vi "SQLite Query - Add New Columns.vi"(8 "error in (no error)":errorcluster, 9 "LV Data Types":T1[](array[typedef]) format="%.0x", 10 "Headers":string[](array[string]), 11 "TableLogger_SQLite_Actor in":refnum<class "TableLogger_SQLite_Actor.lvclass">) -> (0 "error out":errorcluster, 3 "TableLogger_SQLite_Actor out":refnum<class "TableLogger_SQLite_Actor.lvclass">)   [LabVIEW 2014, in "TableLogger_SQLite_Actor.lvlib" / "TableLogger_SQLite_Actor.lvclass"]
uses:
  TableLogger_SQLite_Actor.lvclass
  <userlib>/_OpenG.lib/lvdata/lvdata.llb/Type Descriptor Enumeration__ogtk.ctl
  TableLogger_SQLite_Actor.lvclass/TableLogger_SQLite_Actor.ctl
  <vilib>/drjdpowell/SQLite Library/SQL Connection/Execute SQL.vi
  <userlib>/_OpenG.lib/array/array.llb/Remove Duplicates from 1D Array (String)__ogtk.vi
  <vilib>/drjdpowell/SQLite Library/SQL Connection/Execute SQL (No results).vi
  <vilib>/drjdpowell/SQLite Library/SQLite.lvlib
  <vilib>/drjdpowell/SQLite Library/SQL Connection/Connection.lvclass
panel:
  # "Connector Pane"
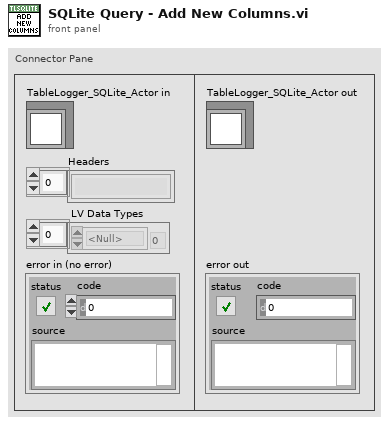
[diagram p1: front panel]
types:
  T1 = typedef "Type Descriptor Enumeration__ogtk.ctl" = enum8{"<Null>", "I8", "I16", "I32", "I64", "U8", "U16", "U32", "U64", "SGL", "DBL", "EXT", "CSG", "CDB", "CXT", "0x0F", "0x10", "0x11", "0x12", "0x13", "0x14", "Enum U8", "Enum U16", "Enum U32", "Enum U64", "SGL PQ", "DBL PQ", "EXT PQ", "CSG PQ", "CDB PQ", "CXT PQ", "0x1F", "0x20", "Boolean", "0x22", "0x23", "0x24", "0x25", "0x26", "0x27", "0x28", "0x29", "0x2A", "0x2B", "0x2C", "0x2D", "0x2E", "0x2F", "String", "0x31", "Path", "Pict", "0x34", "0x35", "0x36", "DAQ", "0x38", "0x39", "0x3A", "0x3B", "0x3C", "0x3D", "0x3E", "0x3F", "Array", "0x41", "0x42", "0x43", "0x44", "0x45", "0x46", "0x47", "0x48", "0x49", "0x4A", "0x4B", "0x4C", "0x4D", "0x4E", "0x4F", "Cluster", "0x51", "0x52", "Variant", "Waveform", "0x55", "0x56", "0x57", "0x58", "0x59", "0x5A", "0x5B", "0x5C", "0x5D", "0x5E", "0x5F", "0x60", "0x61", "0x62", "0x63", "0x64", "0x65", "0x66", "0x67", "0x68", "0x69", "0x6A", "0x6B", "0x6C", "0x6D", "0x6E", "0x6F", "Refnum"}
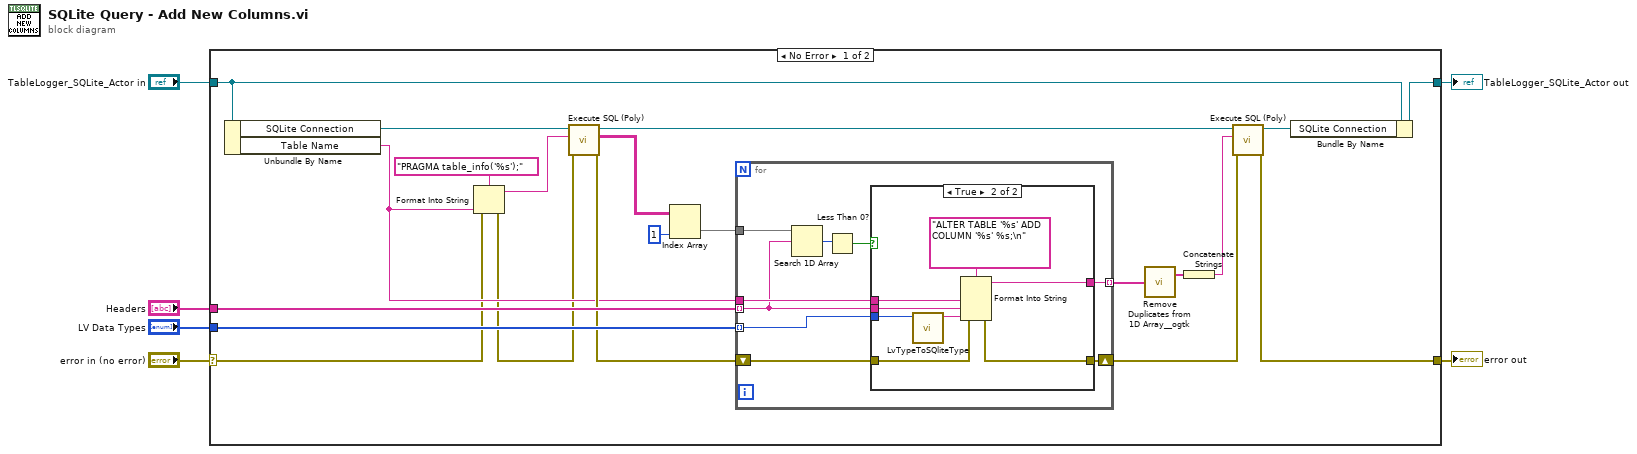
[diagram p0: block diagram]
diagram:
  n1 = case shown="No Error" "error in (no error)" {
    selector: "error in (no error)" -> [w9 w46]
    tunnel: [w26 w47] -> w5
    tunnel: "Headers" -> [w23 _]
    tunnel: "LV Data Types" -> [w21 _]
    tunnel: [w12 w46] -> w4
    tunnel: "TableLogger_SQLite_Actor in" -> [w11 w47]
    frame No Error {
      n2 = Unbundle By Name(w11) -> ("SQLite Connection"=w18:refnum<class "Connection.lvclass">, "Table Name"=w10:string)
      n3 = Format Into String(format string="PRAGMA table_info('%s');" ("SQL"), error in=w9, w10) -> (resulting string=w14:string, error out=w8:errorcluster)  [unwired: 1 in]
      n4 = call-poly <vilib>:"Execute SQL (Poly).vi"("error in (no error)"=w8, "SQL"=w14, "SQLite Connection in"=w18) -> ("error out"=w19:errorcluster, "Result Set"=w15:string[][], "SQLite Connection"=w7:refnum<class "Connection.lvclass">)  [unwired: 5 in, 1 out]
      n5 = Index Array(array=w15, index (col)=1 ("disabled index (col)")) -> (element=w17:string[])  [unwired: 1 in]
      n6 = for {
        tunnel: w17 -> [w36]
        tunnel: w10 -> [w32]
        tunnel: w23 -> [w31] mode=indexing
        shift-right: [w34] -> w20
        shift-left: w19 -> [w35]
        tunnel: w21 -> [w29] mode=indexing
        tunnel: [w28] -> w24 mode=indexing
        n7 = Search 1D Array(1D array=w36, element=w31) -> (index of element=w33:i32)  [unwired: 1 in]
        n8 = Less Than 0?(x=w33) -> (x < 0?=w30:bool)
        n9 = case shown="True" w30 {
          tunnel: w35 -> [w37 w40]
          tunnel: [w37 w39] -> w34
          tunnel: w32 -> [_ w44]
          tunnel: w31 -> [_ w43]
          tunnel: w29 -> [_ w42]
          tunnel: [_ w41] -> w28
          frame False {
          }
          frame True {
            n10 = call "LvTypeToSQliteType.vi"("Type Descriptor Enumeration"=w42) -> ("String"=w38:string)  [unwired: 10 in]
            n11 = Format Into String(format string="ALTER TABLE '%s' ADD COLUMN '%s' %s;\n" ("SQL"), error in=w40, w44, w43, w38) -> (resulting string=w41:string, error out=w39:errorcluster)  [unwired: 1 in]
          }
        }
      }
      n12 = call-poly <userlib>:"Remove Duplicates from 1D Array__ogtk.vi"("Input Array"=w24) -> ("Output Array"=w25:string[])  [unwired: 1 out]
      n13 = Concatenate Strings(w25) -> (w22:string)
      n14 = call-poly <vilib>:"Execute SQL (Poly).vi"("error in (no error)"=w20, "SQL"=w22, "SQLite Connection in"=w7) -> ("error out"=w12:errorcluster, "SQLite Connection"=w27:refnum<class "Connection.lvclass">)  [unwired: 7 in]
      n15 = Bundle By Name(cluster=w11, "SQLite Connection"=w27) -> (w26:refnum<class "TableLogger_SQLite_Actor.lvclass">)
    }
    frame Error {
    }
  }
  "TableLogger_SQLite_Actor out" <- w5
  "error out" <- w4
